vi "Flatten Packet To Message String.vi"(8 "error in (no error)":errorcluster, 10 "Message Packet":variant, 11 "BasicNetworkProtocol in":refnum<class "BasicNetworkProtocol.lvclass">) -> (0 "error out":errorcluster, 3 "Packet as Message String":string)   [LabVIEW 2019, in "Network Logger Examples.lvlib" / "BasicNetworkProtocol.lvclass"]
uses:
  <vilib>/gpm_packages/@cs/event-logger/Examples/Examples/BasicNetworkProtocol/BasicNetworkProtocol.lvclass
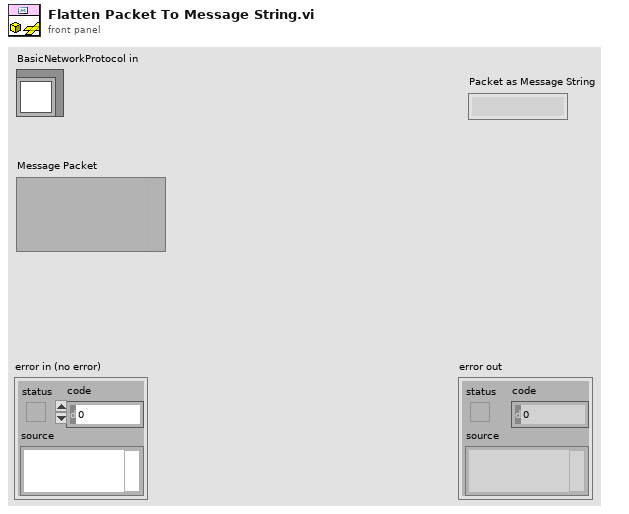
[diagram p1: front panel]
types:
  T1 = cluster{"type string":i16[], "data string":string}
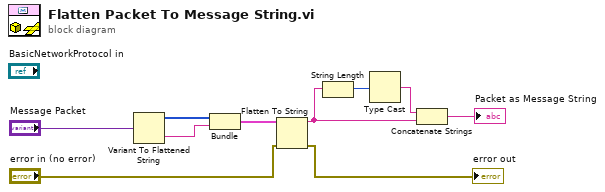
[diagram p0: block diagram]
diagram:
  n1 = Variant To Flattened String(Variant="Message Packet") -> (data string=w8:string, 1:w9:i16[])
  n2 = Bundle("type string"=w9, "data string"=w8) -> (w7:T1)  [unwired: 1 in]
  n3 = Flatten To String(anything=w7, error in (no error)="error in (no error)") -> (data string=w4:string, error out=→"error out":errorcluster)  [unwired: 2 in, 1 out]
  n4 = String Length(string=w4) -> (length=w2:i32)
  n5 = Type Cast(x=w2) -> (*(type *) &x=w3:string)  [unwired: 1 in]
  n6 = Concatenate Strings(w3, w4) -> (→"Packet as Message String":string)
